vi "Compile APU 1.1 Data.vi"(8 "error in (no error)":errorcluster, 11 "Device Item Ref in":T3 format="%.0x") -> (0 "error out":errorcluster, 2 "APUs":T1[](array[typedef]) {"shared settings"."cycle start" format="%#.15g"}, 3 "Device Item Ref out":T3 format="%.0x")   [LabVIEW 2020, in "Engine Simulation Toolkit System Explorer.lvlib"]
uses:
  Engine Simulation Toolkit System Explorer.lvlib
  <vilib>/NI VeriStand/Custom Device API/Custom Device Item Ref.ctl
  Shared/1.1 APU Engine Data.ctl
  Shared/1.0 APU Engine FIFO Idxs.ctl
  DBL Angle to U16.vi
  Shared/Properties.vi
  Shared/Constants and GUIDs.vi
  <vilib>/NI VeriStand/Custom Device Tools/Custom Device Utility Library/NI VeriStand - Search for All Items by GUID.vi
  <vilib>/NI VeriStand/Custom Device API/Get Item Property (String).vi
  <vilib>/NI VeriStand/Custom Device API/Get Item Property (Double).vi
  <vilib>/NI VeriStand/Custom Device API/Get Item Property (Boolean).vi
  <vilib>/NI VeriStand/Custom Device API/Get Item Property (U16).vi
  <vilib>/NI VeriStand/Custom Device Tools/Custom Device Utility Library/NI VeriStand - Search for Item by GUID.vi
  Shared/Engine Simulation Toolkit Shared.lvlib
  <vilib>/NI VeriStand/Custom Device API/Custom Device API.lvlib
  <vilib>/NI VeriStand/Custom Device Tools/Custom Device Utility Library/Custom Device Utility Library.lvlib
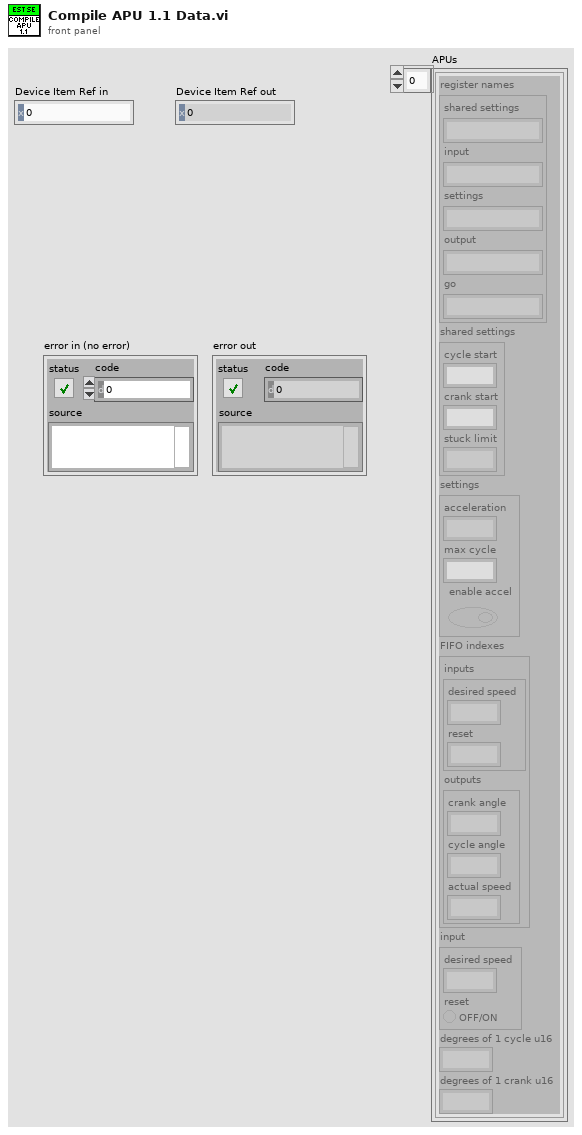
[diagram p1: front panel]
types:
  T1 = typedef "Engine Simulation Toolkit Shared.lvlib/1.1 APU Engine Data.ctl" = cluster{"register names":cluster{"shared settings":string, "input":string, "settings":string, "output":string, "go":string}, "shared settings":cluster{"cycle start":fxp<+,2,2>, "crank start":u16, "stuck limit":fxp<+,18,18>}, "settings":cluster{"acceleration":fxp<+,18,-20>, "max cycle":fxp<+,2,2>, "enable accel":bool}, "FIFO indexes":T2, "input":cluster{"desired speed":fxp<+/-,23,2>, "reset":bool}, "degrees of 1 cycle u16":dbl, "degrees of 1 crank u16":dbl}
  T2 = typedef "Engine Simulation Toolkit Shared.lvlib/1.0 APU Engine FIFO Idxs.ctl" = cluster{"inputs":cluster{"desired speed":i32, "reset":i32}, "outputs":cluster{"crank angle":i32, "cycle angle":i32, "actual speed":i32}}
  T3 = typedef "Custom Device API.lvlib/Custom Device Item Ref.ctl" = u64
  T4 = typedef "Engine Simulation Toolkit Shared.lvlib/Channel.ctl" = cluster{"Name":string, "Units":string, "Default":dbl, "Description":string, "Scalable":bool}
  T5 = cluster{"desired speed":fxp<+/-,23,2>, "reset":bool}
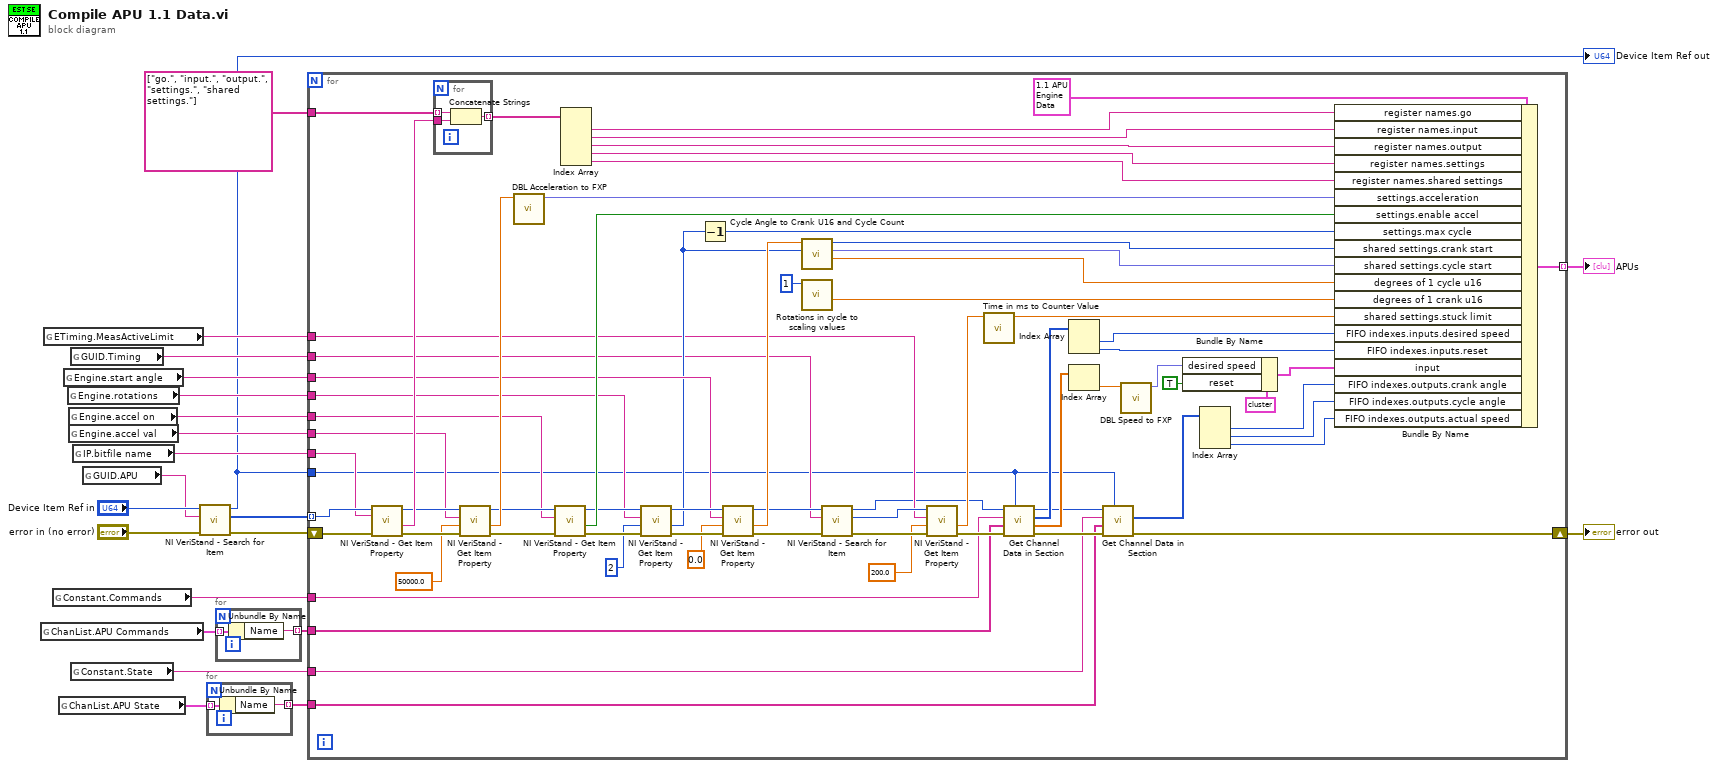
[diagram p0: block diagram]
diagram:
  n1 = global read "Constants and GUIDs.vi" "ChanList.APU Commands"() -> (w5:T4[])
  n2 = global read "Properties.vi" "ETiming.MeasActiveLimit"() -> (w10:string)
  n3 = global read "Constants and GUIDs.vi" "Constant.Commands"() -> (w9:string)
  n4 = global read "Constants and GUIDs.vi" "ChanList.APU State"() -> (w3:T4[])
  n5 = global read "Properties.vi" "Engine.start angle"() -> (w12:string)
  n6 = global read "Properties.vi" "Engine.rotations"() -> (w13:string)
  n7 = global read "Properties.vi" "Engine.accel on"() -> (w14:string)
  n8 = global read "Properties.vi" "Engine.accel val"() -> (w16:string)
  n9 = global read "Constants and GUIDs.vi" "GUID.Timing"() -> (w11:string)
  n10 = global read "Constants and GUIDs.vi" "Constant.State"() -> (w6:string)
  n11 = global read "Properties.vi" "IP.bitfile name"() -> (w18:string)
  n12 = global read "Constants and GUIDs.vi" "GUID.APU"() -> (w20:string)
  n13 = call-poly <vilib>:"NI VeriStand - Search for Item.vi"("error in"="error in (no error)", "Item GUID"=w20, "Section Ref in"="Device Item Ref in") -> ("error out"=w19:errorcluster, "Item Refs"=w1:T3[], "Section Ref out"=w7:T3)  [unwired: 5 in, 1 out]
  "Device Item Ref out" <- w7
  n14 = for {
    tunnel: w3 -> [w24] mode=indexing
    tunnel: [w23] -> w2 mode=indexing
    n15 = Unbundle By Name(w24) -> ("Name"=w23:string)
  }
  n16 = for {
    tunnel: w5 -> [w26] mode=indexing
    tunnel: [w25] -> w4 mode=indexing
    n17 = Unbundle By Name(w26) -> ("Name"=w25:string)
  }
  n18 = for {
    shift-right: [w46] -> w15
    shift-left: w19 -> [w97]
    tunnel: w1 -> [w96] mode=indexing
    tunnel: w18 -> [w95]
    tunnel: string[] ["go.", "input.", "output.", "settings.", "shared settings."] -> [w93]
    tunnel: w16 -> [w88]
    tunnel: w14 -> [w82]
    tunnel: w13 -> [w78]
    tunnel: w12 -> [w74]
    tunnel: w11 -> [w65]
    tunnel: w10 -> [w62]
    tunnel: w9 -> [w57]
    tunnel: w4 -> [w33]
    tunnel: [w51] -> w8 mode=indexing
    tunnel: w7 -> [w45]
    tunnel: w6 -> [w43]
    tunnel: w2 -> [w32]
    n19 = call-poly <vilib>:"NI VeriStand - Get Item Property.vi"("error in (no error)"=w97, "Property Name"=w95, "Item Ref in"=w96) -> ("error out"=w89:errorcluster, "Value"=w94:string, "Item Ref out"=w90:T3)  [unwired: 5 in, 1 out]
    n20 = for {
      tunnel: w94 -> [w100]
      tunnel: w93 -> [w99] mode=indexing
      tunnel: [w98] -> w91 mode=indexing
      n21 = Concatenate Strings(w99, w100) -> (w98:string)
    }
    n22 = call-poly <vilib>:"NI VeriStand - Get Item Property.vi"("error in (no error)"=w89, "Default Value"=50000.0, "Property Name"=w88, "Item Ref in"=w90) -> ("error out"=w87:errorcluster, "Value"=w86:dbl, "Item Ref out"=w83:T3)  [unwired: 4 in, 1 out]
    n23 = call "DBL Acceleration to FXP.vi"("Desired acceleration (RPM/sec)"=w86) -> ("FXP acceleration"=w85:fxp<+,18,-20>)  [unwired: 6 in, 4 out]
    n24 = call-poly <vilib>:"NI VeriStand - Get Item Property.vi"("error in (no error)"=w87, "Property Name"=w82, "Item Ref in"=w83) -> ("error out"=w84:errorcluster, "Value"=w81:bool, "Item Ref out"=w79:T3)  [unwired: 5 in, 1 out]
    n25 = Index Array(array=w91) -> (element #1=w31:string, element #2=w30:string, element #3=w29:string, element #4=w28:string, element #5=w27:string)  [unwired: 5 in]
    n26 = call-poly <vilib>:"NI VeriStand - Get Item Property.vi"("error in (no error)"=w84, "Default Value"=u16 2, "Property Name"=w78, "Item Ref in"=w79) -> ("error out"=w80:errorcluster, "Value"=w70:u16, "Item Ref out"=w75:T3)  [unwired: 4 in, 1 out]
    n27 = Decrement(x=w70) -> (x-1=w37:u16)
    n28 = call-poly <vilib>:"NI VeriStand - Get Item Property.vi"("error in (no error)"=w80, "Default Value"=0.0, "Property Name"=w74, "Item Ref in"=w75) -> ("error out"=w76:errorcluster, "Value"=w71:dbl, "Item Ref out"=w66:T3)  [unwired: 4 in, 1 out]
    n29 = call "Cycle Angle to Crank U16 and Cycle Count.vi"("rotations"=w70, "cycle angle"=w71) -> ("degrees of one u16"=w36:dbl, "cycle count"=w68:fxp<+,2,2>, "crank U16"=w69:u16)  [unwired: 7 in]
    n30 = call "Rotations in cycle to scaling values.vi"("rotations in a cycle"=u16 1) -> ("degrees of one u16"=w34:dbl)  [unwired: 8 in, 2 out]
    n31 = call-poly <vilib>:"NI VeriStand - Search for Item.vi"("error in"=w76, "Item GUID"=w65, "Section Ref in"=w66) -> ("error out"=w67:errorcluster, "Item Ref"=w63:T3, "Section Ref out"=w58:T3)  [unwired: 5 in, 1 out]
    n32 = call-poly <vilib>:"NI VeriStand - Get Item Property.vi"("error in (no error)"=w67, "Default Value"=200.0, "Property Name"=w62, "Item Ref in"=w63) -> ("error out"=w64:errorcluster, "Value"=w60:dbl)  [unwired: 4 in, 2 out]
    n33 = call "Time in ms to Counter Value.vi"("time (ms)"=w60) -> ("counter value"=w59:dbl)  [unwired: 10 in]
    n34 = call "Get Channel Data in Section.vi"("Custom device ref"=w45, "error in (no error)"=w64, "Channels"=w33, "Section (\"\":none)"=w57, "Item Ref in"=w58) -> ("error out"=w56:errorcluster, "default values"=w50:dbl[], "FIFO indexes"=w55:i32[], "Item Ref out"=w44:T3)  [unwired: 2 in, 1 out]
    n35 = Index Array(array=w55) -> (element #1=w54:i32, element #2=w53:i32)  [unwired: 2 in]
    n36 = Index Array(array=w50) -> (element=w49:dbl)  [unwired: 1 in]
    n37 = call "Get Channel Data in Section.vi"("Custom device ref"=w45, "error in (no error)"=w56, "Channels"=w32, "Section (\"\":none)"=w43, "Item Ref in"=w44) -> ("error out"=w46:errorcluster, "FIFO indexes"=w42:i32[])  [unwired: 2 in, 3 out]
    n38 = call "DBL Speed to FXP.vi"("Desired speed (RPM)"=w49) -> ("FXP speed"=w47:fxp<+/-,23,2>)  [unwired: 6 in, 4 out]
    n39 = Bundle By Name(cluster=T5 {"desired speed"=0.0, "reset"=FALSE} ("input"), "desired speed"=w47, "reset"=TRUE) -> (w48:T5)
    n40 = Index Array(array=w42) -> (element #1=w41:i32, element #2=w40:i32, element #3=w39:i32)  [unwired: 3 in]
    n41 = Bundle By Name(cluster=T1 {"register names"={"shared settings"="", "input"="", "settings"="", "output"="", "go"=""}, "shared settings"={"cycle start"=0.0, "crank start"=0, "stuck limit"=0.0}, "settings"={"acceleration"=0.0, "max cycle"=0.0, "enable accel"=FALSE}, "FIFO indexes"={"inputs"={"desired speed"=0, "reset"=0}, "outputs"={"crank angle"=0, "cycle angle"=0, "actual speed"=0}}, "input"={"desired speed"=0.0, "reset"=FALSE}, "degrees of 1 cycle u16"=0.0, "degrees of 1 crank u16"=0.0} ("1.0.0 APU"), "register names.go"=w31, "register names.input"=w30, "register names.output"=w29, "register names.settings"=w28, "register names.shared settings"=w27, "settings.acceleration"=w85, "settings.enable accel"=w81, "settings.max cycle"=w37, "shared settings.crank start"=w69, "shared settings.cycle start"=w68, "degrees of 1 cycle u16"=w36, "degrees of 1 crank u16"=w34, "shared settings.stuck limit"=w59, "FIFO indexes.inputs.desired speed"=w54, "FIFO indexes.inputs.reset"=w53, "input"=w48, "FIFO indexes.outputs.crank angle"=w41, "FIFO indexes.outputs.cycle angle"=w40, "FIFO indexes.outputs.actual speed"=w39) -> (w51:T1)
  }
  "error out" <- w15
  "APUs" <- w8
